vi "TreeMap V1 to V2 recurse.vi"(7 "V2 Map in":T1, 11 "V1":T5(c390)) -> (0 "error out":errorcluster, 5 "V2 Map out":T1)   [LabVIEW 2020, in "Blue Tree Map OpenSource.lvlib"]
uses:
  Blue Tree Map OpenSource.lvlib
  Typedefs/Attribute Map.ctl
  Typedefs/Tree Map.ctl
  Typedefs/Tree Map Data.ctl
  Typedefs/Tree Node Data.ctl
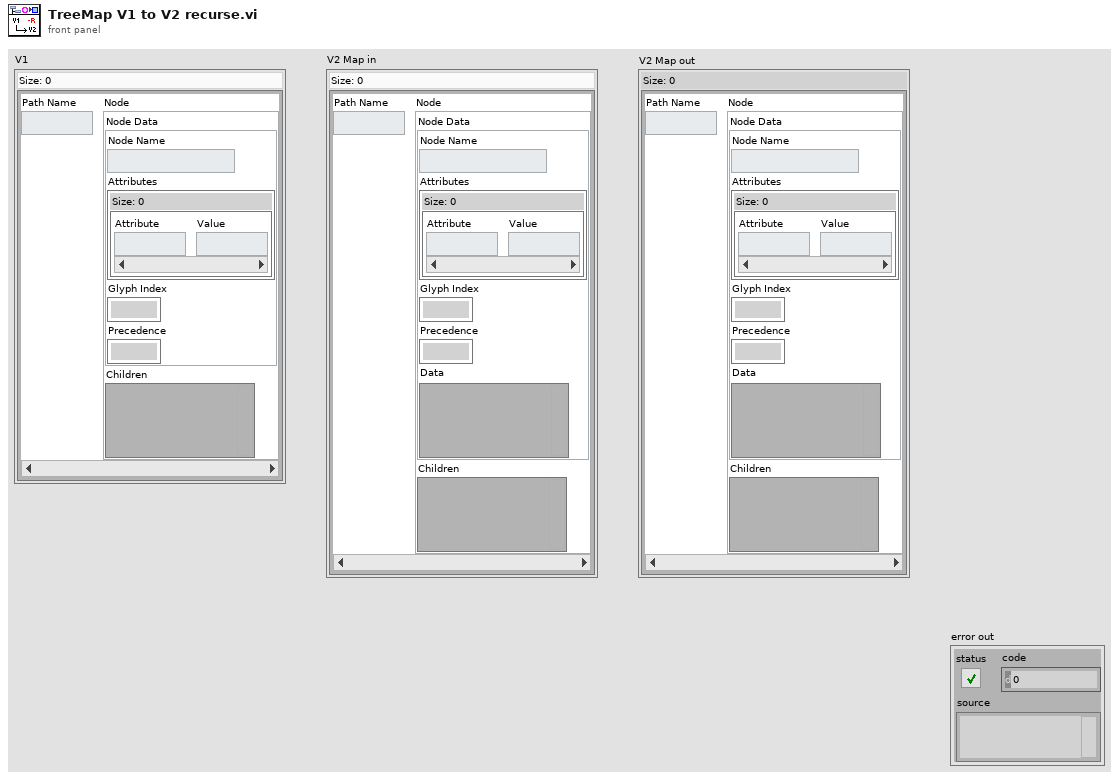
[diagram p1: front panel]
types:
  T1 = typedef "Blue Tree Map OpenSource.lvlib/Tree Map.ctl" = map{string, T2}
  T2 = typedef "Blue Tree Map OpenSource.lvlib/Tree Map Data.ctl" = cluster{"Node Data":T3, "Children":variant}
  T3 = typedef "Blue Tree Map OpenSource.lvlib/Tree Node Data.ctl" = cluster{"Node Name":string, "Attributes":T4, "Glyph Index":i32, "Precedence":i32, "Data":variant}
  T4 = typedef "Blue Tree Map OpenSource.lvlib/Attribute Map.ctl" = map{string, string}
  T5 = map{string, cluster{"Node Data":cluster{"Node Name":string, "Attributes":T4, "Glyph Index":i32, "Precedence":i32}, "Children":variant}}
  T6 = cluster{"Node Data":cluster{"Node Name":string, "Attributes":T4, "Glyph Index":i32, "Precedence":i32}, "Children":variant}
  T7 = cluster{"Node Name":string, "Attributes":T4, "Glyph Index":i32, "Precedence":i32}
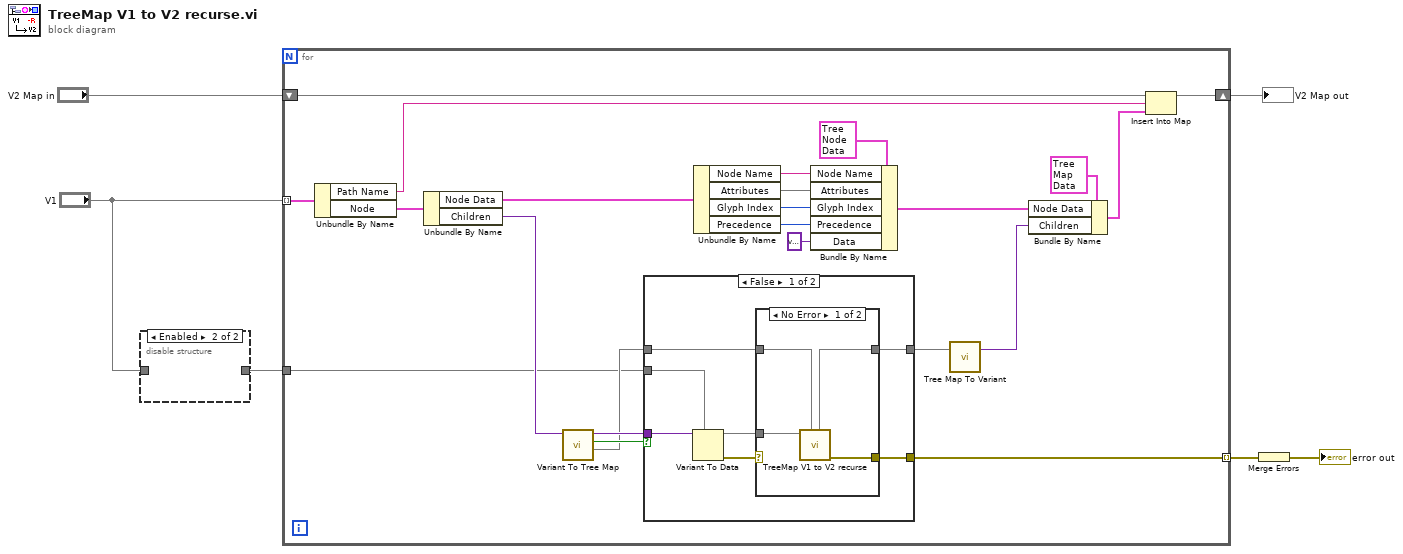
[diagram p0: block diagram]
diagram:
  n1 = disable-structure shown="Enabled" {
    disable-tunnel: "V1" -> [w7 _]
    disable-tunnel: [w7 _] -> w1
    frame Disabled {
    }
    frame Enabled {
    }
  }
  n2 = for {
    tunnel: "V1" -> [w14] mode=indexing
    shift-right: [w19] -> w5
    shift-left: "V2 Map in" -> [w11]
    tunnel: w1 -> [w8]
    tunnel: [w9] -> w4 mode=indexing
    n3 = Unbundle By Name(w14) -> ("Path Name"=w21:string, "Node"=w30:T6)
    n4 = Unbundle By Name(w30) -> ("Node Data"=w15:T7, "Children"=w18:variant)
    n5 = call "Variant To Tree Map.vi"("Children"=w18) -> ("Tree Map (Empty)"=w10:T1, "Empty?"=w17:bool, "Children"=w16:variant)  [unwired: 8 in]
    n6 = case shown="False" w17 {
      tunnel: w16 -> [w37 _]
      tunnel: w8 -> [w36 _]
      tunnel: w10 -> [w33 w44]
      tunnel: [w32 w44] -> w13
      tunnel: [w31 _] -> w9
      frame False {
        n7 = Variant To Data(type=w36, Variant=w37) -> (data=w34:T5, error out=w35:errorcluster)  [unwired: 1 in]
        n8 = case shown="No Error" w35 {
          selector: w35 -> [_ w42]
          tunnel: w34 -> [w41 _]
          tunnel: w33 -> [w40 w43]
          tunnel: [w39 w43] -> w32
          tunnel: [w38 w42] -> w31
          frame No Error {
            n9 = call "TreeMap V1 to V2 recurse.vi"("V2 Map in"=w40, "V1"=w41) -> ("error out"=w38:errorcluster, "V2 Map out"=w39:T1)  [unwired: 8 in]
          }
          frame Error {
          }
        }
      }
      frame True {
      }
    }
    n10 = Unbundle By Name(w15) -> ("Node Name"=w28:string, "Attributes"=w27:T4, "Glyph Index"=w26:i32, "Precedence"=w25:i32)
    n11 = Bundle By Name(cluster=T3 {"Node Name"="", "Attributes"={}, "Glyph Index"=0, "Precedence"=0, "Data"=variant} ("Node Data"), "Node Name"=w28, "Attributes"=w27, "Glyph Index"=w26, "Precedence"=w25, "Data"=variant) -> (w22:T3)
    n12 = call "Tree Map To Variant.vi"("Tree Map"=w13) -> ("Variant"=w12:variant)  [unwired: 2 in]
    n13 = Bundle By Name(cluster=T2 {"Node Data"={"Node Name"="", "Attributes"={}, "Glyph Index"=0, "Precedence"=0, "Data"=variant}, "Children"=variant} ("Node"), "Node Data"=w22, "Children"=w12) -> (w20:T2)
    n14 = Insert Into Map(map in=w11, key=w21, value=w20) -> (map out=w19:T1)  [unwired: 2 out]
  }
  "V2 Map out" <- w5
  n15 = Merge Errors(w4) -> (→"error out":errorcluster)
